vi "ti2_escapeZ.vi"(8 "error in (no error)":errorcluster, 11 "Escape Z":bool) -> (0 "error out":errorcluster)   [LabVIEW 2023, in "ti2lv.lvlib"]
uses:
  ti2lv.lvlib
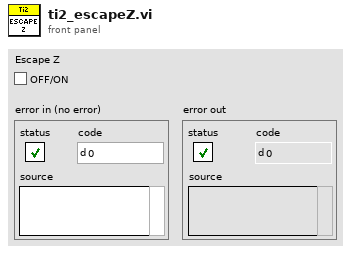
[diagram p1: front panel]
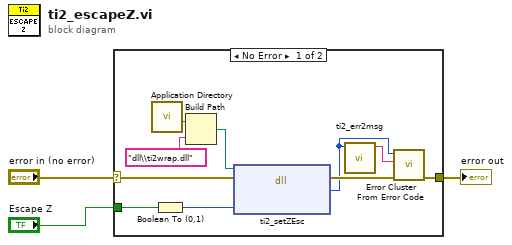
[diagram p0: block diagram]
diagram:
  n1 = case shown="No Error" "error in (no error)" {
    selector: "error in (no error)" -> [w12 w14]
    tunnel: [w13 w14] -> w3
    tunnel: "Escape Z" -> [w5 _]
    frame No Error {
      n2 = call <vilib>:"Application Directory.vi"() -> ("Application Directory"=w7:path)
      n3 = Boolean To (0,1)(Boolean=w5) -> (0, 1=w4:i16)
      n4 = Build Path(base path=w7, name or relative path="dll\\ti2wrap.dll") -> (appended path=w6:path)
      n5 = dll-call lib="C:/FlashGordon/Development/dll/ti2wrap.dll" fn="ti2_setZEsc"(path in=w6, error in=w12, "setting"=w4) -> (error out=w11:errorcluster, "return type"=w10:i32)  [unwired: 2 in, 1 out]
      n6 = call "ti2_err2msg.vi"("Error Code"=w10) -> ("Error Message"=w9:string)  [unwired: 10 in]
      n7 = call <vilib>:"Error Cluster From Error Code.vi"("error in (no error)"=w11, "error message (\"\")"=w9, "error code (0)"=w10) -> ("error out"=w13:errorcluster)  [unwired: 6 in]
    }
    frame Error {
    }
  }
  "error out" <- w3
